vi "Set SSR Status - Multiple.vi"(0 "reference in":refnum<class "SSR.lvclass">, 2 "SSR Channel Number (Zero Based)":i32[](array[numeric]), 4 "SSR Status To Set":bool[](array[boolean]), 5 "error in (no error)":errorcluster) -> (14 "reference out":refnum<class "SSR.lvclass">, 19 "error out":errorcluster)   [LabVIEW 2017, in "SSR.lvclass"]
uses:
  SSR.lvclass
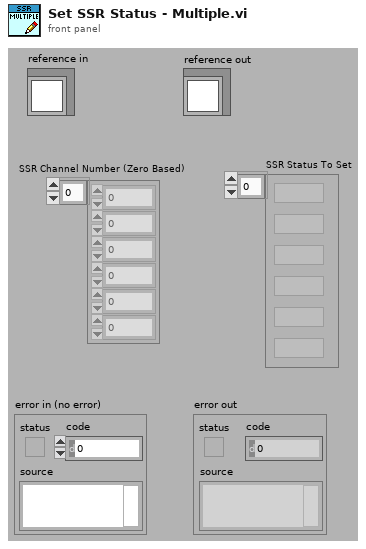
[diagram p1: front panel]
types:
  T1 = typedef "SSR.lvclass/ObjectAttributes.ctl" = cluster{"SSR Task":refnum<k21>, "SSR On/Off Status":bool, "Number of SSR Modules":u32, "Number of Total SSR Channels":u32, "SSR Module Names (NI-Max Name)":string[], "Number of Channels Per SSR Module":i32[], "SSR Status":bool[], "SSR Status to Set":bool[], "SSR VI Reference":refnum<vi>}
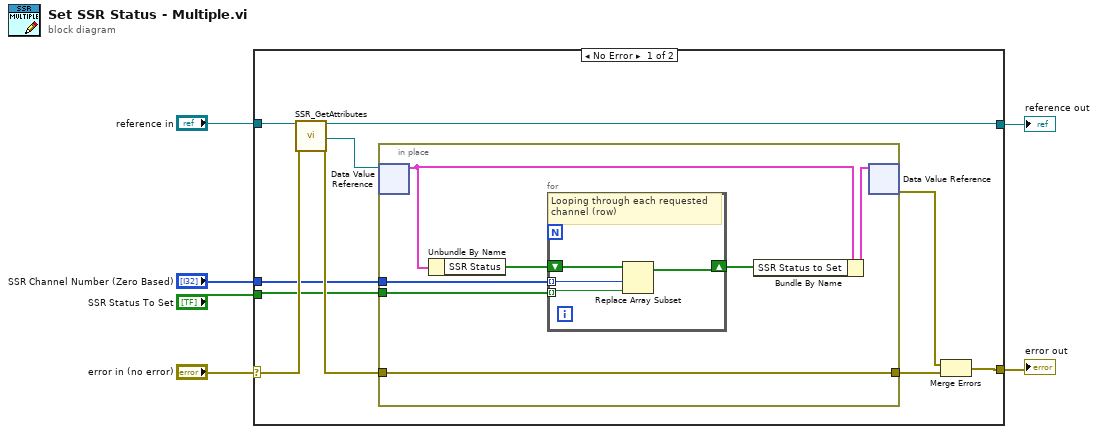
[diagram p0: block diagram]
diagram:
  n1 = case shown="No Error" "error in (no error)" {
    selector: "error in (no error)" -> [w15 w29]
    tunnel: [w12 w29] -> w5
    tunnel: [w13 w28] -> w3
    tunnel: "reference in" -> [w16 w28]
    tunnel: "SSR Channel Number (Zero Based)" -> [w8 _]
    tunnel: "SSR Status To Set" -> [w7 _]
    frame No Error {
      n2 = call "SSR_GetAttributes.vi"("reference in"=w16, "error in (no error)"=w15) -> ("reference out"=w13:refnum<class "SSR.lvclass">, "DataRef"=w11:refnum<data-value>, "error out"=w10:errorcluster)  [unwired: 14 in, 1 out]
      n3 = in-place {
        in-place-border: w10 -> [w21]
        in-place-border: [w21] -> w9
        in-place-border: w8 -> [w18]
        in-place-border: w7 -> [w17]
        n4 = in-place-dvr #1(w11) -> (w22:T1)  [unwired: 1 out]
        n5 = Unbundle By Name(w22) -> ("SSR Status"=w20:bool[])
        n6 = for {
          tunnel: w18 -> [w27] mode=indexing
          tunnel: w17 -> [w26] mode=indexing
          shift-right: [w24] -> w19
          shift-left: w20 -> [w25]
          # "Looping through each requested channel (row)"
          n7 = Replace Array Subset(array=w25, new element=w26, index=w27) -> (w24:bool[])
        }
        n8 = Bundle By Name(cluster=w22, "SSR Status to Set"=w19) -> (w23:T1)
        n9 = in-place-dvr #1(w23) -> (w14:errorcluster)  [unwired: 1 out]
      }
      n10 = Merge Errors(w14, w9) -> (w12:errorcluster)
    }
    frame Error {
    }
  }
  "error out" <- w5
  "reference out" <- w3
